vi "Calc - POIab.vi"(11 "00-00-9220":dbl[](array[numeric])) -> (3 "POIab":dbl)   [LabVIEW 2018, in "Controller (Host).lvlib"]
uses:
  Controller (Host).lvlib
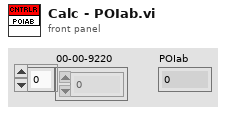
[diagram p1: front panel]
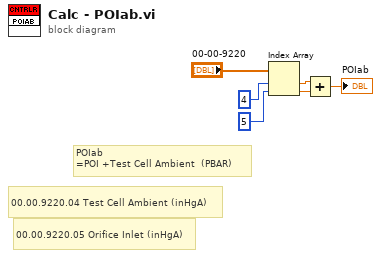
[diagram p0: block diagram]
diagram:
  # "00.00.9220.04\tTest Cell Ambient (inHgA)"
  # "00.00.9220.05\tOrifice Inlet (inHgA)"
  # "POIab\n=POI +Test Cell Ambient  (PBAR)"
  n1 = Index Array(array="00-00-9220", index #1=4 ("index"), index #2=5 ("index")) -> (element #1=w4:dbl, element #2=w5:dbl)
  n2 = Add(x=w4, y=w5) -> (x+y=→"POIab":dbl)
